vi "User Updated Status.vi"(8 "error in (no error)":errorcluster, 10 "Status":string, 11 "Chat Window Model in":refnum<class "Chat Window Model.lvclass">) -> (0 "error out":errorcluster, 3 "Chat Window Model out":refnum<class "Chat Window Model.lvclass">)   [LabVIEW 2020, in "Chat Window Model.lvlib" / "Chat Window Model.lvclass"]
uses:
  Chat Window Model.lvclass
  C:/Program Files/National Instruments/LabVIEW 2020/vi.lib/ActorFramework/Actor/Actor.lvclass
  <vilib>/ActorFramework/Actor/Actor.lvclass/Actor.ctl
  Chat Window Model.lvclass/Chat Window Model.ctl
  Chat Window UI Controller/Chat Window UI Controller Messages/Update VI Title Msg/Update VI Title Msg.lvclass/Update VI Title Msg.ctl
  <vilib>/ActorFramework/Message Enqueuer/Message Enqueuer.lvclass/Message Enqueuer.ctl
  Msg Forward Interface Actor/Msg Forward Interface Actor Messages/Status Updated Msg/Status Updated Msg.lvclass/Status Updated Msg.ctl
  <vilib>/ActorFramework/Message Enqueuer/Enqueue.vi
  Chat Window UI Controller/Chat Window UI Controller Messages/Update VI Title Msg/Update VI Title Msg.lvclass
  C:/Program Files/National Instruments/LabVIEW 2020/vi.lib/ActorFramework/Message/Message.lvclass
  Msg Forward Interface Actor/Msg Forward Interface Actor Messages/Status Updated Msg/Status Updated Msg.lvclass
  <vilib>/ActorFramework/Message Priority Queue/Priority Enqueue.vi
  <vilib>/ActorFramework/Actor/Actor.lvclass
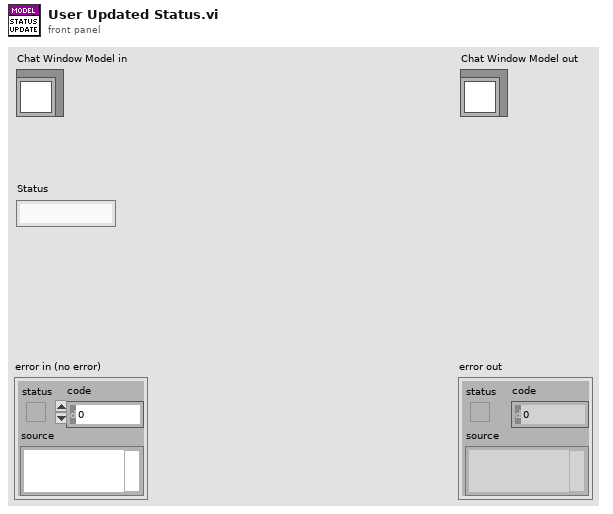
[diagram p1: front panel]
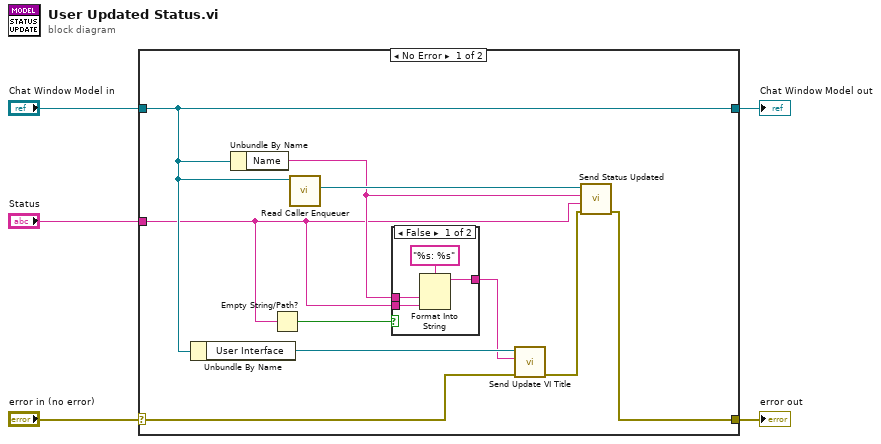
[diagram p0: block diagram]
diagram:
  n1 = case shown="No Error" "error in (no error)" {
    selector: "error in (no error)" -> [w13 w22]
    tunnel: [w6 w22] -> w4
    tunnel: [w15 w21] -> w2
    tunnel: "Chat Window Model in" -> [w15 w21]
    tunnel: "Status" -> [w8 _]
    frame No Error {
      n2 = Unbundle By Name(w15) -> ("User Interface"=w14:refnum<class "Message Enqueuer.lvclass">)
      n3 = Unbundle By Name(w15) -> ("Name"=w9:string)
      n4 = Empty String/Path?(string/path=w8) -> (empty?=w11:bool)
      n5 = call <vilib>:"Read Caller Enqueuer.vi"("Actor"=w15) -> ("Caller Enqueuer"=w10:refnum<class "Message Enqueuer.lvclass">)  [unwired: 10 in]
      n6 = case shown="False" w11 {
        tunnel: [w18 w20] -> w12
        tunnel: w9 -> [w17 w20]
        tunnel: w8 -> [w16 _]
        frame False {
          n7 = Format Into String(format string="%s: %s", w17, w16) -> (resulting string=w18:string)  [unwired: 2 in, 1 out]
        }
        frame True {
        }
      }
      n8 = call "Send Update VI Title.vi"("error in (no error)"=w13, "Window Title"=w12, "Message Enqueuer"=w14) -> ("error out"=w7:errorcluster)  [unwired: 7 in, 1 out]
      n9 = call "Send Status Updated.vi"("error in (no error)"=w7, "Status"=w8, "Name"=w9, "Message Enqueuer"=w10) -> ("error out"=w6:errorcluster)  [unwired: 6 in, 1 out]
    }
    frame Error {
    }
  }
  "error out" <- w4
  "Chat Window Model out" <- w2
